vi "Driver Interface Template.vi"(8 "Error In":errorcluster, 11 "Configuration":T1) -> (0 "Error Out":errorcluster, 3 "PPMS data out":dbl[](array[numeric]))   [LabVIEW 2016]
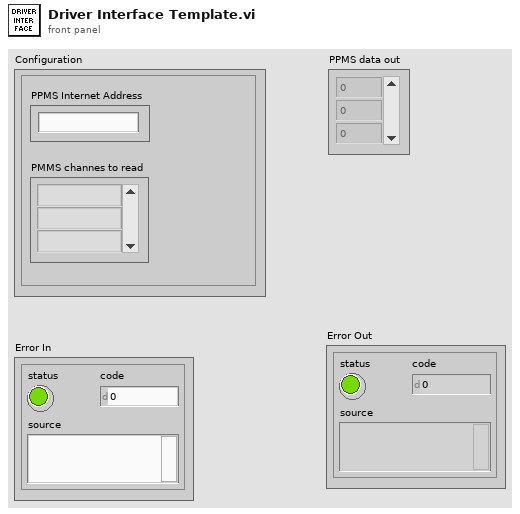
[diagram p1: front panel]
types:
  T1 = cluster{"PPMS Internet Address":string, "PMMS channes to read":string[]}
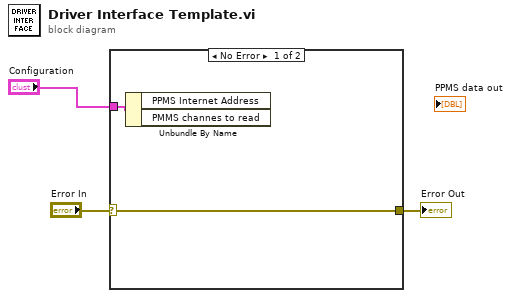
[diagram p0: block diagram]
diagram:
  n1 = case shown="No Error" "Error In" {
    selector: "Error In" -> [w4 w6]
    tunnel: [w4 w6] -> w2
    tunnel: "Configuration" -> [w5 _]
    frame No Error {
      n2 = Unbundle By Name(w5) -> ()  [unwired: 2 out]
    }
    frame Error {
    }
  }
  "Error Out" <- w2
